vi "ApplyTableAppearance.vi"(6 "Defer Updates? (T)":bool=TRUE, 7 "Layout Ref":refnum<vi>, 8 "error in (no error)":errorcluster, 9 "Mode Index":i32=2, 10 "Col Array in":refnum<class "Column.lvclass">[](array[class]), 11 "Table Ref in":refnum<vi>) -> (0 "error out":errorcluster, 3 "Table Ref out":refnum<vi>)   [LabVIEW 2013]
doc: "(Re)Initialize table appearance from column (appearance) array. A layout reference is required so that the existing layout view is preserved. The user can choose not to 'defer panel updates,' although the default is recommended to keep the program responsive."
uses:
  codes/ColumnVIs/Column/Column.lvclass
  <vilib>/Utility/miscctls.llb/LVRowAndColumnTypeDef.ctl
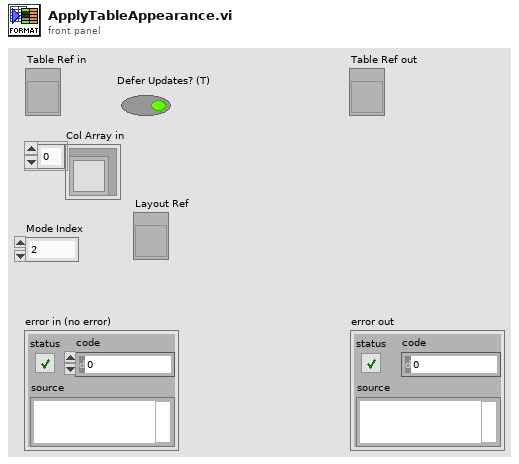
[diagram p1: front panel]
types:
  T1 = typedef "LVRowAndColumnTypeDef.ctl" = cluster{"Row":i32, "Column":i32}
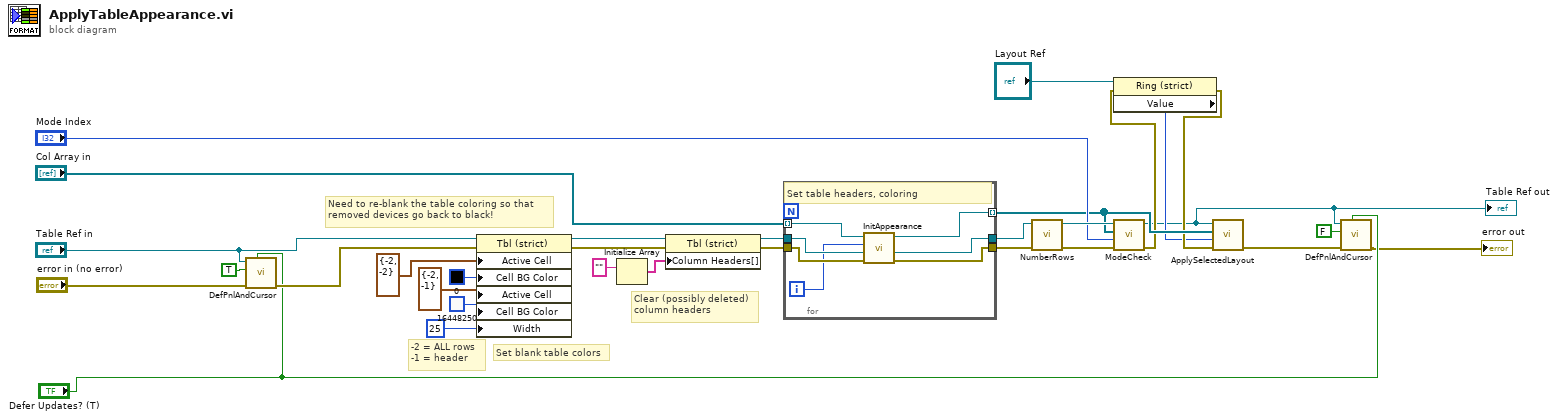
[diagram p0: block diagram]
diagram:
  # "Clear (possibly deleted)\ncolumn headers"
  # "Need to re-blank the table coloring so that\nremoved devices go back to black!"
  # "-2 = ALL rows\n-1 = header"
  # "Set blank table colors"
  n1 = call "DefPnlAndCursor.vi"("AllowDefPan? (T)"="Defer Updates? (T)", "error in (no error)"="error in (no error)", "DeferPanUpdts?"=TRUE, "Tbl Ctrl Refnum"="Table Ref in") -> ("error out"=w9:errorcluster)  [unwired: 7 in]
  n2 = property class="Tbl (strict)"(reference="Table Ref in", error in=w9, "Active Cell"=T1 {"Row"=-2, "Column"=-2} ("RowAndCollumn"), "Cell BG Color"=u32 0, "Active Cell"=T1 {"Row"=-2, "Column"=-1} ("RowAndCollumn"), "Cell BG Color"=u32 16448250, "Width"=u32 25 ("Active Cell:Cell Size:Width")) -> (reference out=w15:refnum<vi>, error out=w13:errorcluster)
  n3 = Initialize Array("") -> (w10:string[])  [unwired: 1 in]
  n4 = property class="Tbl (strict)"(reference=w15, error in=w13, "Column Headers[]"=w10) -> (reference out=w14:refnum<vi>, error out=w12:errorcluster)
  n5 = for {
    tunnel: "Col Array in" -> [w33] mode=indexing
    tunnel: [w37] -> w30
    tunnel: w12 -> [w38]
    tunnel: w14 -> [w35]
    tunnel: [w36] -> w31
    tunnel: [w32] -> w20 mode=indexing
    i -> [w34]
    # "Set table headers, coloring"
    n6 = call-dynamic "InitAppearance.vi"("error in (no error)"=w38, "Table Ref in"=w35, "Col #"=w34, "Column in"=w33) -> ("error out"=w37:errorcluster, "Table Ref out"=w36:refnum<vi>, "Column out"=w32:refnum<class "Column.lvclass">)  [unwired: 5 in]
  }
  n7 = call "NumberRows.vi"("error in (no error)"=w30, "Table Ref in"=w31) -> ("error out"=w29:errorcluster, "Table Ref out"=w28:refnum<vi>)  [unwired: 8 in]
  n8 = call "ModeCheck.vi"("error in (no error)"=w29, "mode col. index"="Mode Index", "Col Array in"=w20, "Table Ref in"=w28) -> ("error out"=w18:errorcluster, "Table Ref out"=w4:refnum<vi>)  [unwired: 6 in]
  "Table Ref out" <- w4
  n9 = property class="Ring (strict)"(reference="Layout Ref", error in=w18) -> (error out=w17:errorcluster, "Value"=w16:i32)  [unwired: 1 out]
  n10 = call "ApplySelectedLayout.vi"("error in (no error)"=w17, "Layout index"=w16, "Col array"=w20, "Tbl Refnum"=w4) -> ("error out"=w5:errorcluster)  [unwired: 7 in]
  n11 = call "DefPnlAndCursor.vi"("AllowDefPan? (T)"="Defer Updates? (T)", "error in (no error)"=w5, "DeferPanUpdts?"=FALSE, "Tbl Ctrl Refnum"=w4) -> ("error out"=→"error out":errorcluster)  [unwired: 7 in]
